vi "DHTRead.vi"(8 "Error In":errorcluster, 10 "DHT Data Pin":u8, 11 "LINX Resource":T1) -> (0 "Error Out":errorcluster, 2 "DHT Readings":T7, 3 "LINX Resource":T1)   [LabVIEW 2014, in "LMH-LINX.lvlib" / "Interaction Parts Kit.lvlib"]
doc: "Reads data from the DHT11."
uses:
  <vilib>/MakerHub/LINX/Public/Sensors/Digilent/Interaction Parts Kit/Interaction Parts Kit.lvlib
  <vilib>/MakerHub/LINX/Private/Type Defs/LINX Ref.ctl
  <vilib>/MakerHub/LINX/Private/Type Defs/Platform.ctl
  <vilib>/MakerHub/LINX/Private/Type Defs/Interface.ctl
  <vilib>/MakerHub/LINX/Private/Device/Type Defs/LINX Device Config.ctl
  <vilib>/MakerHub/LINX/Private/Device/Type Defs/TCP Config.ctl
  <vilib>/MakerHub/LINX/Private/Device/Type Defs/Channels.ctl
  <vilib>/MakerHub/LINX/LMH-LINX.lvlib
  <vilib>/MakerHub/LINX/Private/Device/Device.lvlib
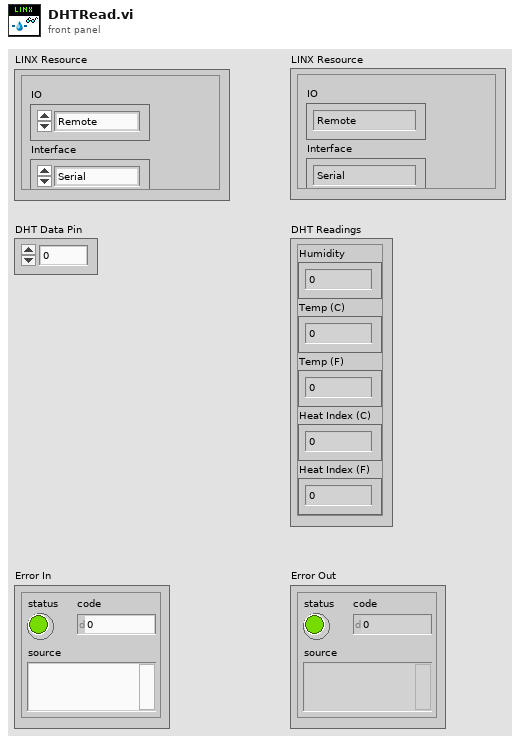
[diagram p1: front panel]
types:
  T1 = typedef "LMH-LINX.lvlib/LINX Ref.ctl" = cluster{"IO":T2, "Interface":T3, "LINX Device Config":T4}
  T2 = typedef "LMH-LINX.lvlib/Platform.ctl" = enum16{"Remote", "Local"}
  T3 = typedef "LMH-LINX.lvlib/Interface.ctl" = enum16{"Serial", "TCP"}
  T4 = typedef "LMH-LINX.lvlib/Device.lvlib/LINX Device Config.ctl" = cluster{"Interface":T3, "COM Port":refnum<visa-resource-name>, "TCP Configuration":T5, "Device Family":u8, "Device ID":u8, "Device Name":string, "TCP Ref":refnum<k5>, "Channels":T6}
  T5 = typedef "LMH-LINX.lvlib/Device.lvlib/TCP Config.ctl" = cluster{"IP Address":string, "Port":u16}
  T6 = typedef "LMH-LINX.lvlib/Channels.ctl" = cluster{"DI":u8[], "DO":u8[], "AI":u8[], "AO":u8[], "PWM":u8[], "QE":u8[], "UART":u8[], "I2C 2":u8[], "SPI":u8[], "CAN":u8[], "Servo":u8[], "AI Ref (V)":dbl, "AI Resolution (Bits)":u8, "AO Ref (V)":dbl, "AO Resolution (Bits)":u8}
  T7 = cluster{"Humidity":u8, "Temp (C)":u8, "Temp (F)":u8, "Heat Index (C)":u8, "Heat Index (F)":u8}
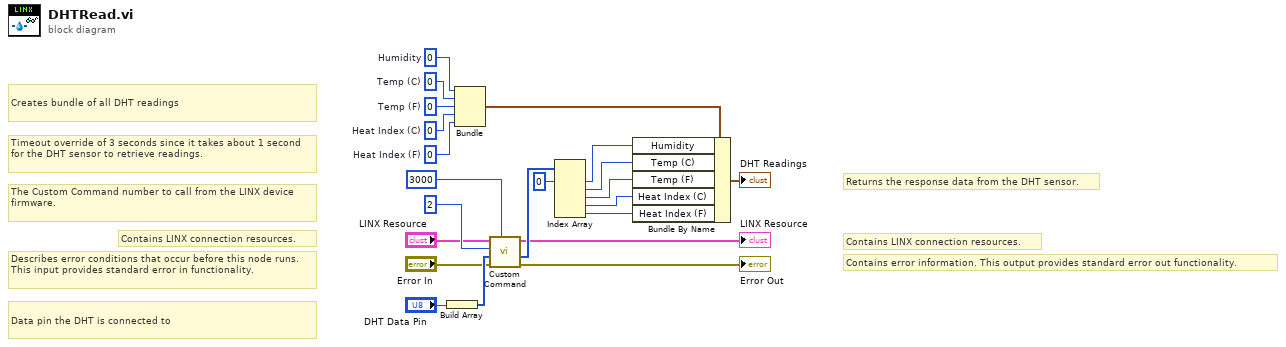
[diagram p0: block diagram]
diagram:
  w14 = u8 0  # Heat Index (F)
  w15 = u8 0  # Heat Index (C)
  w16 = u8 0  # Temp (F)
  w17 = u8 0  # Temp (C)
  w18 = u8 0  # Humidity
  # "Timeout override of 3 seconds since it takes about 1 second for the DHT sensor to retrieve readings."
  # "Data pin the DHT is connected to"
  # "Creates bundle of all DHT readings"
  # "The Custom Command number to call from the LINX device firmware."
  # "Returns the response data from the DHT sensor."
  # "Contains LINX connection resources."
  # "Contains error information. This output provides standard error out functionality."
  # "Contains LINX connection resources."
  # "Describes error conditions that occur before this node runs. This input provides standard error in functionality."
  n1 = Build Array("DHT Data Pin") -> (w5:u8[])
  n2 = Bundle("Humidity"=w18, "Temp (C)"=w17, "Temp (F)"=w16, "Heat Index (C)"=w15, "Heat Index (F)"=w14) -> (w13:T7)  [unwired: 1 in]
  n3 = call <vilib>:"Custom Command.vi"("Timeout (100 ms)"=3000, "Error In"="Error In", "Data"=w5, "Custom Command Number"=u16 2, "LINX Resource"="LINX Resource") -> ("Error Out"=→"Error Out":errorcluster, "Response"=w20:u8[], "LINX Resource"=→"LINX Resource":T1)  [unwired: 3 in, 1 out]
  n4 = Index Array(array=w20, index #1=0 ("index")) -> (element #1=w12:u8, element #2=w11:u8, element #3=w10:u8, element #4=w9:u8, element #5=w8:u8)  [unwired: 4 in]
  n5 = Bundle By Name(cluster=w13, "Humidity"=w12, "Temp (C)"=w11, "Temp (F)"=w10, "Heat Index (C)"=w9, "Heat Index (F)"=w8) -> (→"DHT Readings":T7)
